vi "Save_DistParts.vi"(8 "error in (no error)":errorcluster, 11 "Class in":refnum<class "IB_MSI.lvclass">) -> (0 "error out":errorcluster, 3 "Class out":refnum<class "IB_MSI.lvclass">)   [LabVIEW 2020, in "IB_MSI.lvclass"]
uses:
  <vilib>/AppBuilder/IB_Classes/MSI/IB_MSI.lvclass
  <vilib>/AppBuilder/IB_Classes/MSI/IB_MSI.lvclass/IB_MSI.ctl
  <vilib>/AppBuilder/IB_Classes/DistPart/IB_DistPart.lvclass
  <vilib>/AppBuilder/IB_Classes/Installer/Installer.lvclass
  e:/builds/penguin/labview/branches/2020/dev/dist/vi.lib/AppBuilder/IB_Classes/Installer/Installer.lvclass
  e:/builds/penguin/labview/branches/2020/dev/dist/vi.lib/AppBuilder/IB_Classes/MSI/IB_MSI.lvclass
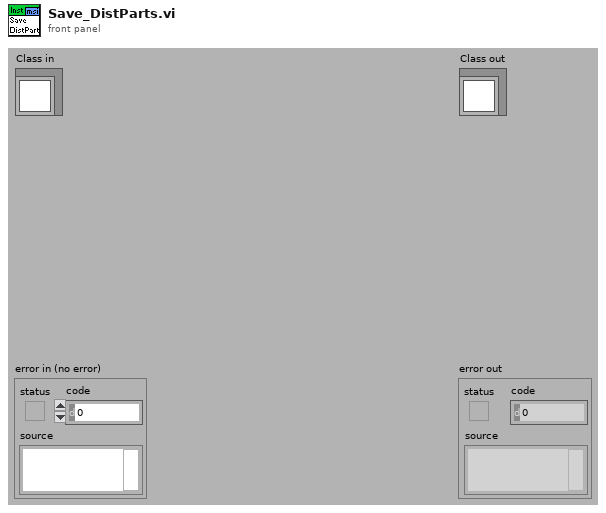
[diagram p1: front panel]
types:
  T1 = typedef "IB_Installer.ctl" = cluster{"Destination":refnum<class "IB_Destination.lvclass">[], "Source":refnum<class "IB_Source.lvclass">[], "buildObject":T2, "defaultDir":string, "platform":string, "author":string, "productName":string, "buildSpecName":string, "hide":bool, "requireLVDevSys":bool, "autoIncrement":bool, "includeError":bool, "readmeID":string, "buildLocation":path, "readmePath":path, "mediaSize":u16, "language":T3, "productVersion":T4, "preview":bool, "programmatic":bool, "progressBarEvents":T5, "userLog_Path":path, "shortcutAddresses":T7[], "EXE_Install Address":string, "EXE_Uninstall Address":string, "additional NIPaths":refnum<class "Dest_NI_NIPath.lvclass">[], "web service itemIDs":string[], "installerName":string}
  T2 = typedef "ItemRef.ctl" = u64
  T3 = typedef "CDK_sTypeDef_Languages.ctl" = u16
  T4 = typedef "CDK_sTypeDef_ProductVersion.ctl" = cluster{"Major":u8, "Minor":u8, "Update":u16}
  T5 = typedef "provcom_ProgressBar_Events.ctl" = cluster{"newJob":refnum<user-event>, "newItem":refnum<user-event>, "errorMsg":T6, "cancel":refnum<user-event>}
  T6 = typedef "mxLvBuildError.ctl" = refnum<user-event>
  T7 = typedef "CDK_sTypeDef_ShortcutAddress.ctl" = cluster{"file":string, "shortcut":string}
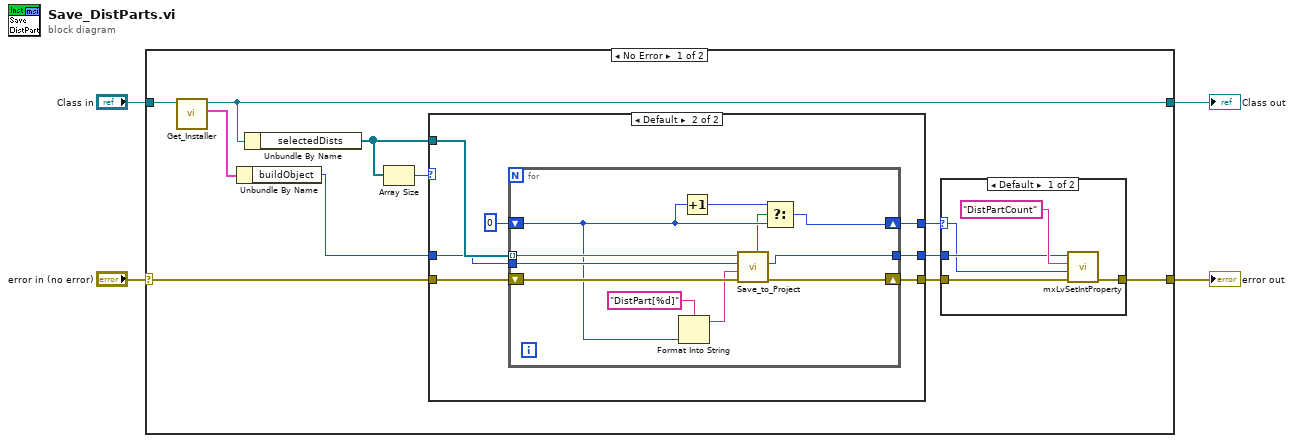
[diagram p0: block diagram]
diagram:
  n1 = case shown="No Error" "error in (no error)" {
    selector: "error in (no error)" -> [w14 w43]
    tunnel: [w13 w43] -> w3
    tunnel: [w15 w42] -> w1
    tunnel: "Class in" -> [w12 w42]
    frame No Error {
      n2 = call <vilib>:"Get_Installer.vi"("Installer in"=w12) -> ("data"=w10:T1, "Installer out"=w15:refnum<class "IB_MSI.lvclass">)  [unwired: 1 in, 8 out]
      n3 = Unbundle By Name(w10) -> ("buildObject"=w9:T2)
      n4 = Unbundle By Name(w15) -> ("selectedDists"=w11:refnum<class "IB_DistPart.lvclass">[])
      n5 = Array Size(array=w11) -> (size(s)=w8:i32)
      n6 = case shown="Default" w8 {
        tunnel: w11 -> [_ w30]
        tunnel: [w23 w29] -> w7
        tunnel: w9 -> [w22 w26]
        tunnel: w14 -> [w23 w25]
        tunnel: [_ w27] -> w6
        tunnel: [w22 w24] -> w5
        frame 0 {
        }
        frame Default {
          n7 = for {
            tunnel: w30 -> [w41] mode=indexing
            tunnel: w26 -> [w40]
            shift-right: [w39] -> w29
            shift-left: w25 -> [w38]
            shift-right: [w36] -> w27
            shift-left: 0 -> [w37]
            tunnel: [w31] -> w24
            n8 = Format Into String(format string="DistPart[%d]", w37) -> (resulting string=w34:string)  [unwired: 2 in, 1 out]
            n9 = Increment(x=w37) -> (x+1=w33:i32)
            n10 = call <vilib>:"Save_to_Project.vi"("error in (no error)"=w38, "index"=w34, "buildObject"=w40, "Class in"=w41) -> ("error out"=w39:errorcluster, "buildObject out"=w31:T2, "saved?"=w32:bool)  [unwired: 5 out]
            n11 = Select(t=w33, s=w32, f=w37) -> (s? t:f=w36:i32)
          }
        }
      }
      n12 = case shown="Default" w6 {
        selector: w6 -> [w16 _]
        tunnel: [w18 w21] -> w13
        tunnel: w7 -> [w19 w21]
        tunnel: w5 -> [w17 _]
        frame Default {
          n13 = call <resource>:"mxLvSetIntProperty.vi"("error in"=w19, "Value (0)"=w16, "Tag"="DistPartCount", "Item"=w17) -> ("error out"=w18:errorcluster)  [unwired: 1 in, 6 out]
        }
        frame 0 {
        }
      }
    }
    frame Error {
    }
  }
  "error out" <- w3
  "Class out" <- w1
